vi "Leer_2.vi"() -> ()   [LabVIEW 2016]
panel:
  out "text 2":string[](array[string])
  out "text":string
  in  "file path (use dialog)":path
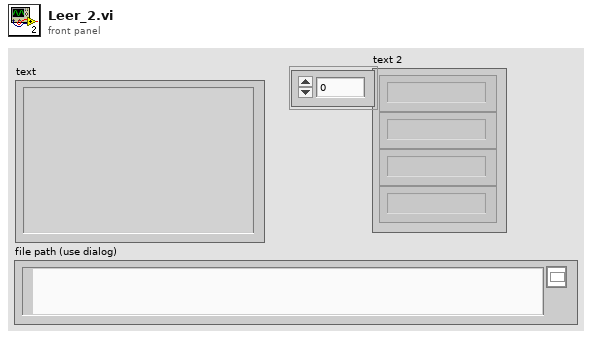
[diagram p1: front panel]
types:
  T1 = enum16{"open", "replace", "create", "open or create", "replace or create", "replace or create with confirmation"}
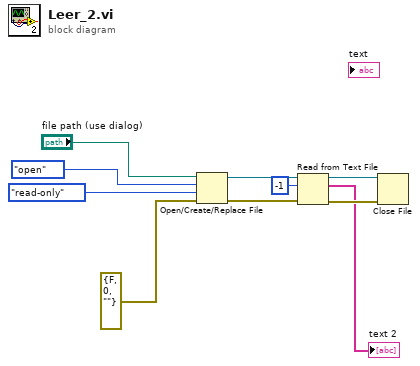
[diagram p0: block diagram]
diagram:
  n1 = Open/Create/Replace File(file path (use dialog)="file path (use dialog)", error in=errorcluster {"status"=FALSE, "code"=0, "source"=""}, operation (0:open)=T1."open", access (0:read/write)=enum16{"read/write", "read-only", "write-only"}."read-only") -> (refnum out=w6:refnum<file>, error out=w5:errorcluster)  [unwired: 2 in, 1 out]
  n2 = Read from Text File(file (use dialog)=w6, count=-1, error in=w5) -> (refnum out=w3:refnum<file>, text=→"text 2":string[], error out=w2:errorcluster)  [unwired: 1 in, 1 out]
  n3 = Close File(refnum=w3, error in=w2) -> ()  [unwired: 2 out]
